vi "feedback-positive_negative.vi"(7 "callee":refnum<vi>, 8 "error in (no error)":errorcluster, 10 "dialog_text_fail":string, 11 "dialog_text_success":string) -> (0 "error out":errorcluster)   [LabVIEW 2015, in "lv-dialog.lvlib"]
doc: "This will provide positive feedback if no error is wired in and will provide negative feedback if an error is wired in."
uses:
  lv-dialog.lvlib
  api/v1/public/class/v1.lvclass
  api/v1/v1.lvlib
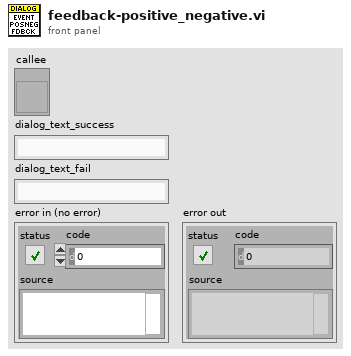
[diagram p1: front panel]
types:
  T1 = cluster{"dialog_text":string, "boolean_text_1":string}
  T2 = cluster{"dialog_text":string, "boolean_text_1":string, "boolean_text_2":string}
  T3 = typedef "lv-dialog.lvlib/v1.lvlib/selection.ctl" = enum16{"null", "panel_closed", "button_1", "button_2", "button_3", "cancelled"}
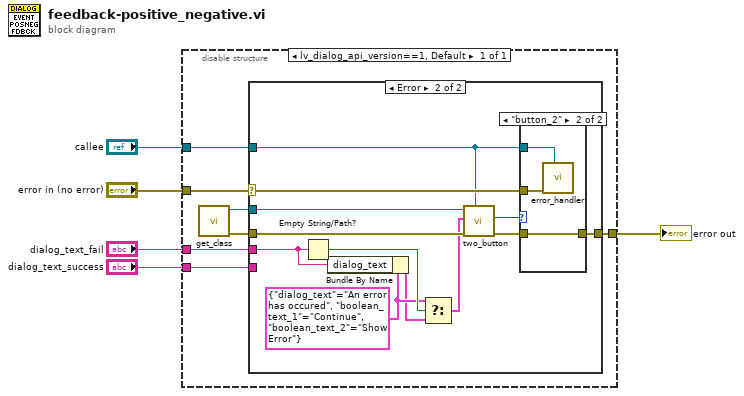
[diagram p0: block diagram]
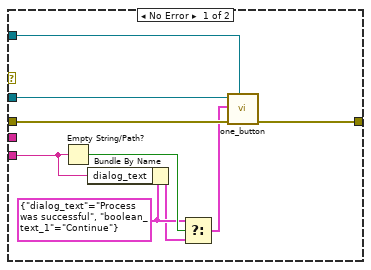
[diagram p2: hidden frame]
diagram:
  n1 = disable-structure shown="lv_dialog_api_version==1, Default" {
    disable-tunnel: "callee" -> [w12]
    disable-tunnel: [w11] -> w2
    disable-tunnel: "error in (no error)" -> [w10]
    disable-tunnel: "dialog_text_fail" -> [w7]
    disable-tunnel: "dialog_text_success" -> [w6]
    frame condition #0 (active) {
      n2 = call "get_class.vi"() -> ("error out"=w9:errorcluster, "class"=w8:refnum<class "v1.lvclass">)  [unwired: 10 in]
      n3 = case shown="Error" w10 {
        selector: w10 -> [_ w30]
        tunnel: w12 -> [w16 w28]
        tunnel: [w18 w31] -> w11
        tunnel: w9 -> [w19 w29]
        tunnel: w8 -> [w17 w27]
        tunnel: w7 -> [_ w24]
        tunnel: w6 -> [w20 _]
        frame No Error {
          w14 = T1 {"dialog_text"="Process was successful", "boolean_text_1"="Continue"} ("configuration")
          n4 = Empty String/Path?(string/path=w20) -> (empty?=w21:bool)
          n5 = Bundle By Name(cluster=w14, "dialog_text"=w20) -> (w13:T1)
          n6 = Select(t=w14, s=w21, f=w13) -> (s? t:f=w15:T1)
          n7 = call-dynamic "one_button.vi"("callee"=w16, "error in (no error)"=w19, "configuration"=w15, "v1 in"=w17) -> ("error out"=w18:errorcluster)  [unwired: 5 in, 2 out]
        }
        frame Error {
          w23 = T2 {"dialog_text"="An error has occured", "boolean_text_1"="Continue", "boolean_text_2"="Show Error"} ("configuration")
          n8 = Empty String/Path?(string/path=w24) -> (empty?=w26:bool)
          n9 = Bundle By Name(cluster=w23, "dialog_text"=w24) -> (w22:T2)
          n10 = Select(t=w23, s=w26, f=w22) -> (s? t:f=w25:T2)
          n11 = call-dynamic "two_button.vi"("callee"=w28, "error in (no error)"=w29, "configuration"=w25, "v1 in"=w27) -> ("error out"=w32:errorcluster, "dialog_selection"=w33:T3)  [unwired: 5 in, 1 out]
          n12 = case shown="\"button_2\"" w33 {
            tunnel: w30 -> [_ w35]
            tunnel: w32 -> [w34 w37]
            tunnel: [w34 w37] -> w31
            tunnel: w28 -> [_ w36]
            frame Default {
            }
            frame "button_2" {
              n13 = call "error_handler.vi"("calling_vi"=w36, "error in (no error)"=w35) -> ()  [unwired: 9 in, 1 out]
            }
          }
        }
      }
    }
  }
  "error out" <- w2
